vi "SN Table Operate_VNA.vi"(0 "Function":enum16{"Query", "Update"}(ring), 5 "Product Type":string(combo)="SFP+", 7 "Day in":string="1", 9 "Tail in":string="1", 11 "SN In":string="0000000001") -> (4 "Day":string="1", 6 "Tail":string="1", 8 "SN_OUT":string="0000000001")   [LabVIEW 2011]
uses:
  <vilib>/addons/database/Connection.llb/DB Tools Open Connec (String).vi
  <vilib>/addons/database/_DB Variant To Data/Database Variant To Data.xnode
  <vilib>/addons/database/NI_Database_API.lvlib
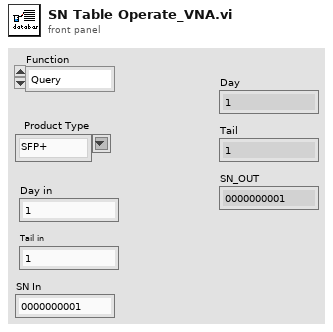
[diagram p1: front panel]
types:
  T1 = cluster{"Day in":string, "Tail in":string, "SN In":string}
  T2 = typedef "NI_Database_API.lvlib/Conn ObjectReference.ctl" = refnum<k1>
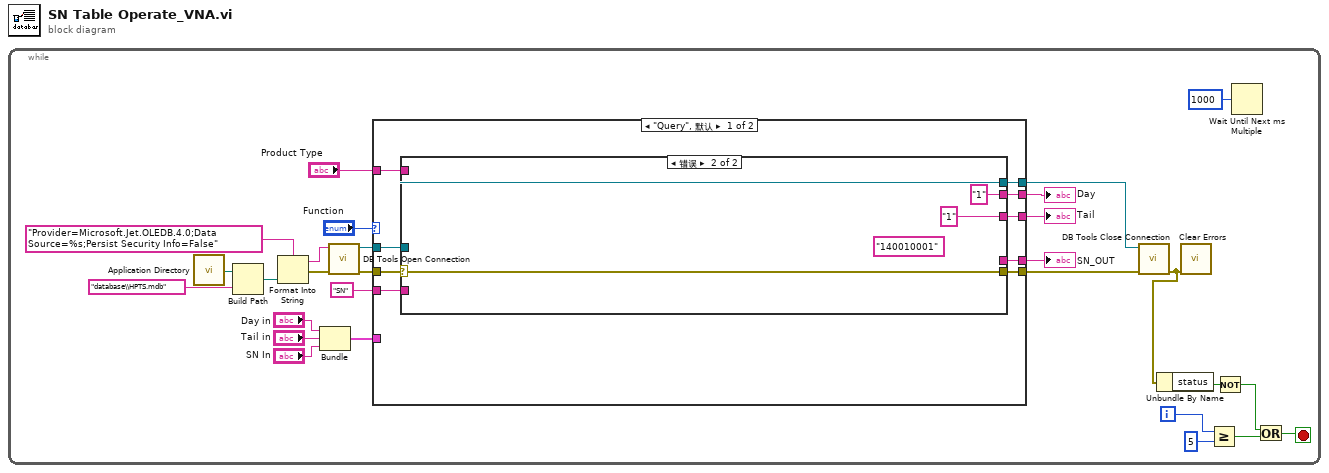
[diagram p0: block diagram]
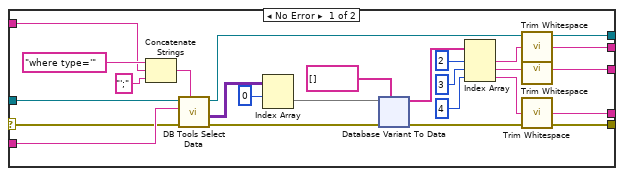
[diagram p2: hidden frame]
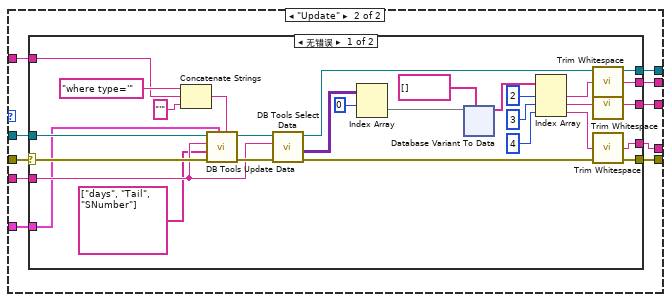
[diagram p3: hidden frame]
diagram:
  n1 = while {
    i -> [w3]
    stop <- w5 stop-if-true
    n2 = call <vilib>:"Application Directory.vi"() -> ("Application Directory"=w28:path)
    n3 = Build Path(base path=w28, name or relative path="database\\HPTS.mdb" ("名称或相对路径")) -> (appended path=w26:path)
    n4 = Format Into String(format string="Provider=Microsoft.Jet.OLEDB.4.0;Data Source=%s;Persist Security Info=False" ("格式字符串"), w26) -> (resulting string=w25:string, error out=w24:errorcluster)  [unwired: 2 in]
    n5 = Bundle("Day in"="Day in", "Tail in"="Tail in", "SN In"="SN In") -> (w18:T1)  [unwired: 1 in]
    n6 = call-poly <vilib>:"DB Tools Open Connection.vi"("error in (no error)"=w24, "connection information"=w25) -> ("error out"=w22:errorcluster, "connection reference"=w21:T2)  [unwired: 6 in]
    n7 = case shown="\"Query\", 默认" "Function" {
      tunnel: "SN" ("table") -> [w37 w110]
      tunnel: w22 -> [w36 w106]
      tunnel: w21 -> [w35 w111]
      tunnel: "Product Type" -> [w34 w112]
      tunnel: w18 -> [_ w113]
      tunnel: [w33 w109] -> w17
      tunnel: [w32 w108] -> w16
      tunnel: [w31 w107] -> w15
      tunnel: [w30 w105] -> w10
      tunnel: [w29 w104] -> w9
      frame "Query", Default {
        n8 = case shown="错误" w36 {
          selector: w36 -> [w58 w100]
          tunnel: w35 -> [w57 w101]
          tunnel: w37 -> [w59 _]
          tunnel: [w52 "1" ("trimmed string")] -> w33
          tunnel: w34 -> [w50 _]
          tunnel: [w42 "1" ("trimmed string")] -> w32
          tunnel: [w41 _] -> w31
          tunnel: [w40 w101] -> w30
          tunnel: [w38 w100] -> w29
          frame No Error {
            n9 = Concatenate Strings("where type='" ("Command Text"), w50, "';" ("字符串")) -> (w48:string)
            n10 = call <vilib>:"DB Tools Select Data.vi"("condition"=w48, "error in (no error)"=w58, "table"=w59, "connection reference"=w57) -> ("error out"=w39:errorcluster, "data"=w56:variant[][], "connection reference out"=w40:T2)  [unwired: 2 in]
            n11 = Index Array(array=w56, index (row)=0 ("禁用的索引 (列)")) -> (element=w60:variant[])  [unwired: 1 in]
            n12 = xnode "Database Variant To Data"("database variant"=w60, "error in"=w39, "type"=string[] []) -> ("data"=w55:string[], "error out"=w38:errorcluster)
            n13 = Index Array(array=w55, index #1=2 ("索引"), index #2=3 ("索引"), index #3=4 ("索引")) -> (element #1=w53:string, element #2=w44:string, element #3=w43:string)
            n14 = call <vilib>:"Trim Whitespace.vi"("string"=w53) -> ("trimmed string"=w52:string)  [unwired: 1 in]
            n15 = call <vilib>:"Trim Whitespace.vi"("string"=w44) -> ("trimmed string"=w42:string)  [unwired: 1 in]
            n16 = call <vilib>:"Trim Whitespace.vi"("string"=w43) -> ("trimmed string"=w41:string)  [unwired: 1 in]
          }
          frame Error {
            (unwired) "140010001" ("trimmed string")
          }
        }
      }
      frame "Update" {
        n17 = case shown="无错误" w106 {
          selector: w106 -> [w136 w180]
          tunnel: [w140 w179] -> w105
          tunnel: [w139 w180] -> w104
          tunnel: w111 -> [w135 w179]
          tunnel: w110 -> [w134 _]
          tunnel: w113 -> [w117 _]
          tunnel: w112 -> [w118 _]
          tunnel: [w123 _] -> w109
          tunnel: [w122 _] -> w108
          tunnel: [w121 _] -> w107
          frame No Error {
            n18 = Concatenate Strings("where type='" ("Command Text"), w118, "'" ("字符串")) -> (w116:string)
            n19 = call <vilib>:"DB Tools Update Data.vi"("condition"=w116, "data"=w117, "error in (no error)"=w136, "columns"=string[] ["days", "Tail", "SNumber"], "table"=w134, "connection reference"=w135) -> ("error out"=w137:errorcluster, "connection reference out"=w138:T2)  [unwired: 4 in]
            n20 = call <vilib>:"DB Tools Select Data.vi"("error in (no error)"=w137, "table"=w134, "connection reference"=w138) -> ("error out"=w139:errorcluster, "data"=w131:variant[][], "connection reference out"=w140:T2)  [unwired: 3 in]
            n21 = Index Array(array=w131, index (row)=0 ("禁用的索引 (列)")) -> (element=w132:variant[])  [unwired: 1 in]
            n22 = xnode "Database Variant To Data"("database variant"=w132, "type"=string[] []) -> ("data"=w124:string[])  [unwired: 1 in, 1 out]
            n23 = Index Array(array=w124, index #1=2 ("索引"), index #2=3 ("索引"), index #3=4 ("索引")) -> (element #1=w129:string, element #2=w126:string, element #3=w125:string)
            n24 = call <vilib>:"Trim Whitespace.vi"("string"=w129) -> ("trimmed string"=w123:string)  [unwired: 1 in]
            n25 = call <vilib>:"Trim Whitespace.vi"("string"=w126) -> ("trimmed string"=w122:string)  [unwired: 1 in]
            n26 = call <vilib>:"Trim Whitespace.vi"("string"=w125) -> ("trimmed string"=w121:string)  [unwired: 1 in]
          }
          frame Error {
          }
        }
      }
    }
    "Day" <- w17
    "SN_OUT" <- w15
    "Tail" <- w16
    n27 = call <vilib>:"DB Tools Close Connection.vi"("error in (no error)"=w9, "connection reference"=w10) -> ("error out"=w8:errorcluster)  [unwired: 5 in]
    n28 = Unbundle By Name(w8) -> ("status"=w7:bool)
    n29 = call <vilib>:"Clear Errors.vi"("error in (no error)"=w8) -> ()  [unwired: 6 in, 1 out]
    n30 = Greater Or Equal?(x=w3, y=5) -> (x >= y?=w4:bool)
    n31 = Not(x=w7) -> (.not. x?=w6:bool)
    n32 = Wait Until Next ms Multiple(millisecond multiple=u32 1000 ("等待时间（毫秒）")) -> ()  [unwired: 1 out]
    n33 = Or(x=w6, y=w4) -> (x .or. y?=w5:bool)
  }
